vi "Temperature_stabil.vi"(5 "error in":errorcluster) -> (4 "error out":errorcluster)   [LabVIEW 2010]
panel:
  in  "TemperatureIn":T1
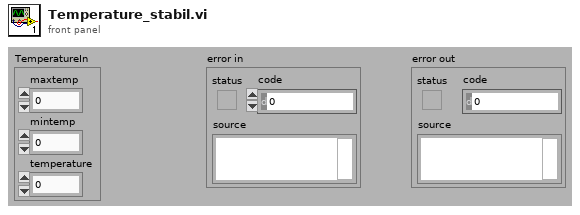
[diagram p1: front panel]
types:
  T1 = cluster{"maxtemp":i32, "mintemp":i32, "temperature":i32}
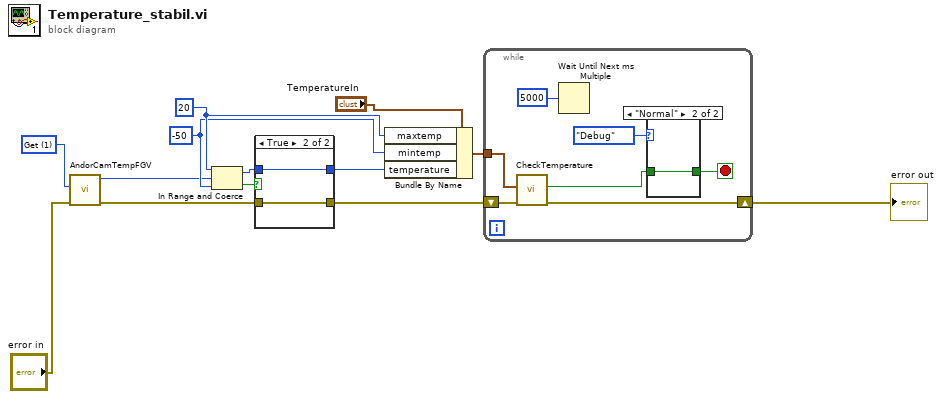
[diagram p0: block diagram]
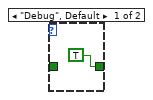
[diagram p2: hidden frame]
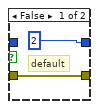
[diagram p3: hidden frame]
diagram:
  w5 = u16 1 items=["Set", "Get"] ("Set_Get")
  w8 = -50 ("mintemp")
  w9 = 20 ("maxtemp")
  n1 = call "AndorCamTempFGV.vi"("error in"="error in", "Set_Get"=w5) -> ("error out"=w3:errorcluster, "TempOut"=w4:i32)  [unwired: 8 in]
  n2 = In Range and Coerce(upper limit=w9, x=w4, lower limit=w8) -> (coerced(x)=w6:i32, In Range?=w7:bool)
  n3 = case shown="True" w7 {
    tunnel: [2 ("mintemp") w17] -> w10
    tunnel: w6 -> [_ w17]
    tunnel: w3 -> [w14 w16]
    tunnel: [w14 w16] -> w1
    frame False {
      # "default"
    }
    frame True {
    }
  }
  n4 = Bundle By Name(cluster="TemperatureIn", "maxtemp"=w9, "mintemp"=w8, "temperature"=w10) -> (w11:T1)
  n5 = while {
    tunnel: w11 -> [w24]
    shift-right: [w21] -> w13
    shift-left: w1 -> [w23]
    stop <- w19 stop-if-true
    n6 = call "CheckTemperature.vi"("error in (no error)"=w23, 10:w24) -> ("error out"=w21:errorcluster, "TemperatureReached"=w18:bool)  [unwired: 7 in, 1 out]
    n7 = Wait Until Next ms Multiple(millisecond multiple=u32 5000) -> ()  [unwired: 1 out]
    n8 = case shown="\"Normal\"" enum16{"Debug", "Normal"}."Debug" {
      tunnel: [TRUE w26] -> w19
      tunnel: w18 -> [_ w26]
      frame "Debug", Default {
      }
      frame "Normal" {
      }
    }
  }
  "error out" <- w13
